vi "Close Panel.vi"(8 "error in (no error)":errorcluster, 10 "ArrayPanel":refnum<class "ArrayPanel.lvclass">, 11 "ArrayManager in":refnum<class "ArrayManager.lvclass">) -> (0 "error out":errorcluster, 3 "ArrayManager out":refnum<class "ArrayManager.lvclass">)   [LabVIEW 2020, in "OOPanel.lvlib" / "ArrayManager.lvclass"]
uses:
  ArrayManager.lvclass
  ArrayManager.lvclass/ArrayManager.ctl
  Manager/Manager.lvclass
  ArrayPanel/ArrayPanel.lvclass
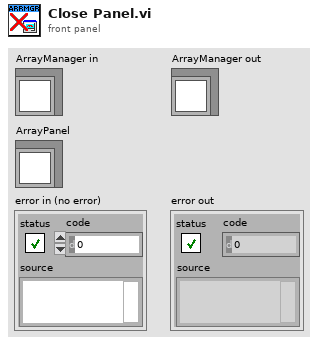
[diagram p1: front panel]
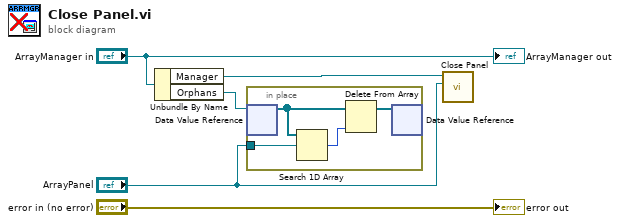
[diagram p0: block diagram]
diagram:
  n1 = Unbundle By Name("ArrayManager in") -> ("Manager"=w2:refnum<class "Manager.lvclass">, "Orphans"=w4:refnum<data-value>)
  n2 = in-place {
    in-place-border: "ArrayPanel" -> [w9]
    n3 = in-place-dvr #1(w4) -> (w8:refnum<class "ArrayPanel.lvclass">[])  [unwired: 1 out]
    n4 = Search 1D Array(1D array=w8, element=w9) -> (index of element=w7:i32)  [unwired: 1 in]
    n5 = Delete From Array(array=w8, index=w7) -> (array with subset deleted=w6:refnum<class "ArrayPanel.lvclass">[])  [unwired: 1 in, 1 out]
    n6 = in-place-dvr #1(w6) -> ()  [unwired: 2 out]
  }
  n7 = call "Close Panel.vi"("Panel"="ArrayPanel", "Manager in"=w2) -> ()  [unwired: 8 in, 2 out]
  "error out" <- "error in (no error)"
  "ArrayManager out" <- "ArrayManager in"
